vi "Host Key Hash.vi"(8 "Error In":errorcluster) -> (0 "Error Out":errorcluster)   [LabVIEW 2017, in "Tests.lvlib" / "Session.lvlib"]
uses:
  Session.lvlib
  src/LabSSH2/Public/Session/Public/Typedefs/Host Key Hash Types.ctl
  src/LabSSH2/LabSSH2.lvlib
  src/LabSSH2/Public/Session/Session.lvclass
  <vilib>/addons/_JKI Toolkits/Caraya/classes/Test/Test.lvclass
  <vilib>/addons/_JKI Toolkits/Caraya/classes/Assert/Assert.lvclass
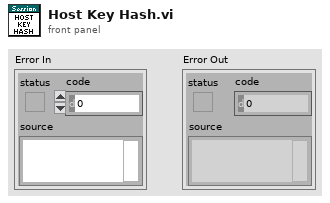
[diagram p1: front panel]
types:
  T1 = typedef "LabSSH2.lvlib/Session.lvclass/Host Key Hash Types.ctl" = enum16{"MD5", "SHA1"}
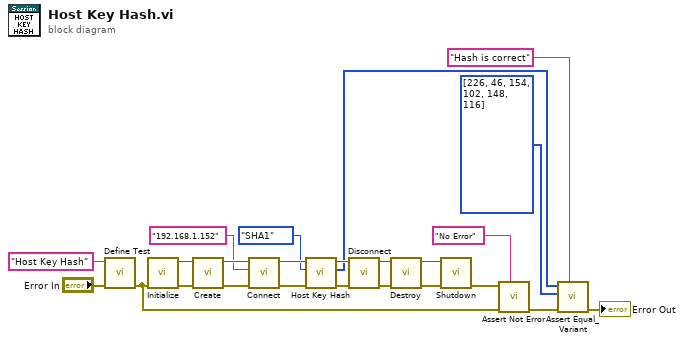
[diagram p0: block diagram]
diagram:
  n1 = call <vilib>:"Define Test.vi"("error in (no error)"="Error In", "Label (VI Title)"="Host Key Hash") -> ("error out"=w19:errorcluster)  [unwired: 9 in]
  n2 = call "Initialize.vi"("Error In"=w19) -> ("Error Out"=w23:errorcluster, "labssh2 Shared Library Out"=w15:path)  [unwired: 9 in]
  n3 = call "Create.vi"("Error In"=w23, "labssh2 Shared Library"=w15) -> ("Error Out"=w13:errorcluster, "Sesssion"=w14:refnum<class "Session.lvclass">)  [unwired: 8 in]
  n4 = call "Connect.vi"("Error In"=w13, "Address"="192.168.1.152", "Session In"=w14) -> ("Error Out"=w6:errorcluster, "Sesssion Out"=w9:refnum<class "Session.lvclass">)  [unwired: 7 in]
  n5 = call "Host Key Hash.vi"("Error In"=w6, "Type"=Host_Key_Hash_Types."SHA1", "Session In"=w9) -> ("Error Out"=w7:errorcluster, "Hash"=w3:u8[], "Sesssion Out"=w8:refnum<class "Session.lvclass">)  [unwired: 6 in]
  n6 = call "Disconnect.vi"("Error In"=w7, "Session In"=w8) -> ("Error Out"=w11:errorcluster, "Sesssion Out"=w12:refnum<class "Session.lvclass">)  [unwired: 8 in]
  n7 = call "Destroy.vi"("Error In"=w11, "Session"=w12) -> ("Error Out"=w21:errorcluster, "labssh2 Shared Library"=w22:path)  [unwired: 8 in]
  n8 = call "Shutdown.vi"("Error In"=w21, "labssh2 Shared Library"=w22) -> ("Error Out"=w20:errorcluster)  [unwired: 9 in]
  n9 = call <vilib>:"Assert Not Error.vi"("Label"="No Error", "error in (no error)"=w19, "Not Error?"=w20) -> ("error out"=w18:errorcluster)  [unwired: 8 in]
  n10 = call <vilib>:"Assert Equal_Variant.vi"("Label"="Hash is correct", "error in (no error)"=w18, "Y"=u8[] [226, 46, 154, 102, 148, 116] ("Fingerprint"), "X"=w3) -> ("error out"=→"Error Out":errorcluster)  [unwired: 7 in]
